vi "TIO RPC Notification U32.vi"(5 "Read":bool, 7 "error in (no error)":errorcluster, 8 "Set value":u32, 9 "Topic":string, 10 "TIO":T1={"TS Connection"={"Type"=enum."Serial", "URL"="serial:///dev/cu.usbserial-00000", "TO"=500, "Addr"=0, "Port"=0, "TCP"=refnum, "UDP"=refnum, "Route"=""}, "REQ"=refnum, "REP"=refnum}) -> (0 "error out":errorcluster, 1 "Get value (default if error)":u32, 2 "Response":bool)   [LabVIEW 2019]
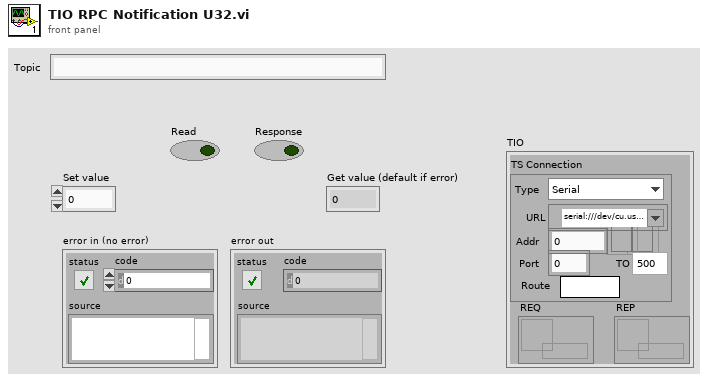
[diagram p1: front panel]
types:
  T1 = cluster{"TS Connection":cluster{"Type":enum16{"Serial", "TCP", "UDP", "mUDP"}, "URL":refnum<visa-resource-name>, "TO":u32, "Addr":u32, "Port":i32, "TCP":refnum<k5>, "UDP":refnum<k16>, "Route":string}, "REQ":refnum<queue>, "REP":refnum<queue>}
  T2 = enum16{"big-endian, network order", "native, host order", "little-endian"}
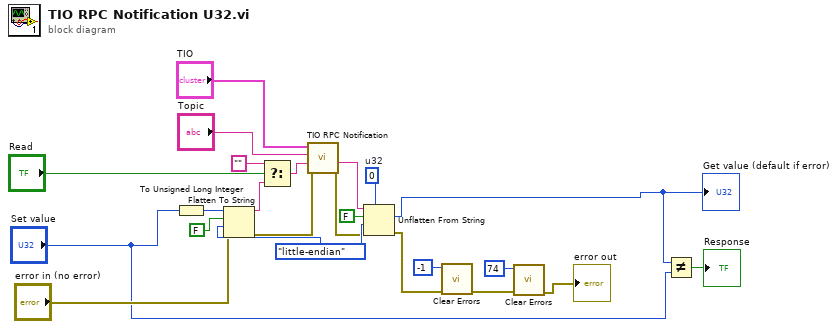
[diagram p0: block diagram]
diagram:
  w23 = u32 0  # u32
  w21 = T2."little-endian" ("byte order (0:big-endian, network order)")
  n1 = To Unsigned Long Integer(number="Set value") -> (unsigned 32bit integer=w17:u32)
  n2 = Flatten To String(anything=w17, prepend array or string size? (T)=FALSE, byte order (0:big-endian, network order)=w21, error in (no error)="error in (no error)") -> (data string=w18:string, error out=w14:errorcluster)  [unwired: 1 out]
  n3 = Select(t="", s="Read", f=w18) -> (s? t:f=w4:string)
  n4 = call "TIO RPC Notification.vi"("error in (no error)"=w14, "Payload"=w4, "Topic"="Topic", "TIO"="TIO") -> ("error out"=w6:errorcluster, "REP"=w1:string)  [unwired: 4 in, 1 out]
  n5 = Unflatten From String(type=w23, binary string=w1, data includes array or string size? (T)=FALSE, byte order (0:big-endian, network order)=w21, error in (no error)=w6) -> (value=w5:u32, error out=w7:errorcluster)  [unwired: 1 out]
  "Get value (default if error)" <- w5
  n6 = call <vilib>:"Clear Errors.vi"("error in (no error)"=w7, "specific error code to clear (0: all)"=-1) -> ("error out"=w12:errorcluster)  [unwired: 4 in, 1 out]
  n7 = call <vilib>:"Clear Errors.vi"("error in (no error)"=w12, "specific error code to clear (0: all)"=74) -> ("error out"=→"error out":errorcluster)  [unwired: 4 in, 1 out]
  n8 = Not Equal?(x=w5, y="Set value") -> (x != y?=→"Response":bool)
